vi "Start Discovery Service.vi"(8 "error in":errorcluster, 11 "key file path":path) -> (0 "error out":errorcluster)   [LabVIEW 2020, in "MeasurementLink Discovery.lvlib"]
doc: "This VI starts the MeasurementLink.DiscoveryService.exe."
uses:
  <vilib>/Utility/sysdir.llb/System Directory Type.ctl
  MeasurementLink Measurement Server/Helpers/Error Strings Global Internal.vi
  <vilib>/ErrorRing/Error Ring.xnode
  MeasurementLink Discovery.lvlib
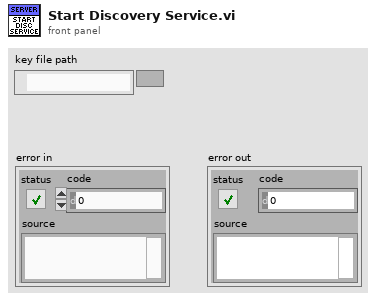
[diagram p1: front panel]
types:
  T1 = enum16{"open", "replace", "create", "open or create", "replace or create", "replace or create with confirmation"}
  T2 = typedef "System Directory Type.ctl" = i32
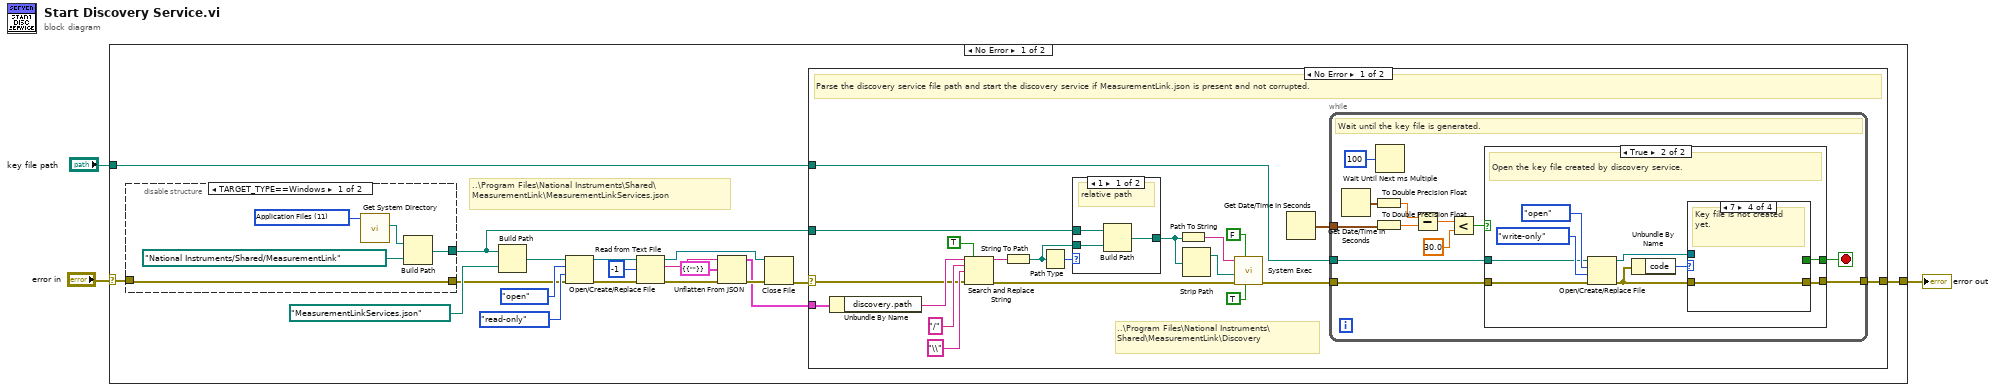
[diagram p0: block diagram]
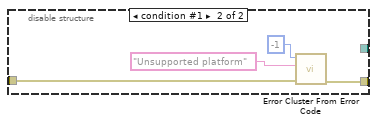
[diagram p2: hidden frame]
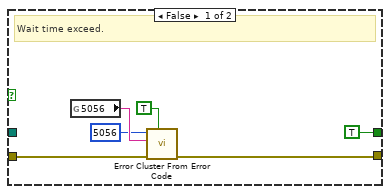
[diagram p4: hidden frame]
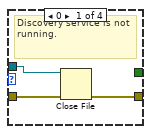
[diagram p5: hidden frame]
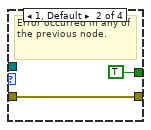
[diagram p6: hidden frame]
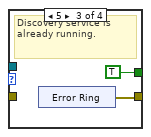
[diagram p7: hidden frame]
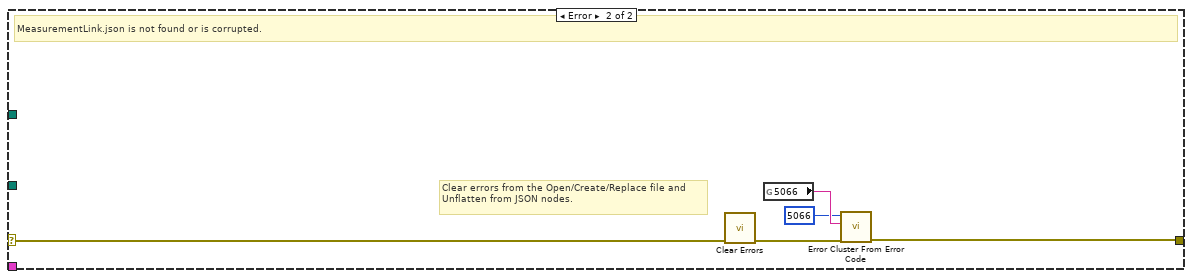
[diagram p8: hidden frame]
diagram:
  n1 = case shown="No Error" "error in" {
    selector: "error in" -> [w17 w97]
    tunnel: [w16 w97] -> w2
    tunnel: "key file path" -> [w15 _]
    frame No Error {
      # "..\\Program Files\\National Instruments\\Shared\\MeasurementLink\\MeasurementLinkServices.json"
      n2 = disable-structure shown="TARGET_TYPE==Windows" {
        disable-tunnel: [w24 _] -> w14
        disable-tunnel: w17 -> [w23 w29]
        disable-tunnel: [w23 w28] -> w18
        frame condition #0 (active) {
          w27 = T2 11 items=["User Home"=0, "User Desktop"=1, "User Documents"=2, "User Application Data"=3, "User Preferences"=4, "User Temporary"=5, "Public Documents"=6, "Public Application Data"=7, "Public Preferences"=8, "Public Cache"=13, "System Core Libraries"=9, "System Installed Libraries"=10, "Application Files"=11, "Boot Volume Root"=12] ("system directory type")
          n3 = call <vilib>:"Get System Directory.vi"("system directory type"=w27) -> ("system directory"=w26:path)  [unwired: 10 in]
          n4 = Build Path(base path=w26, name or relative path=path "National Instruments/Shared/MeasurementLink") -> (appended path=w24:path)
        }
        frame condition #1 {
          n5 = call <vilib>:"Error Cluster From Error Code.vi"("error in (no error)"=w29, "error message (\"\")"="Unsupported platform" ("error message (\"\")"), "error code (0)"=-1) -> ("error out"=w28:errorcluster)  [unwired: 6 in]
        }
      }
      n6 = Build Path(base path=w14, name or relative path=path "MeasurementLinkServices.json") -> (appended path=w21:path)
      n7 = Open/Create/Replace File(file path (use dialog)=w21, error in=w18, operation (0:open)=T1."open", access (0:read/write)=enum16{"read/write", "read-only", "write-only"}."read-only") -> (refnum out=w6:refnum<file>, error out=w9:errorcluster)  [unwired: 2 in, 1 out]
      n8 = Read from Text File(file (use dialog)=w6, count=-1, error in=w9) -> (refnum out=w7:refnum<file>, text=w11:string, error out=w13:errorcluster)  [unwired: 1 in, 1 out]
      n9 = Unflatten From JSON(JSON string=w11, type and defaults=cluster{"discovery":cluster{"path":string}} {"discovery"={"path"=""}}, error in (no error)=w13) -> (value=w4:cluster{"discovery":cluster{"path":string}}, error out=w8:errorcluster)  [unwired: 4 in]
      n10 = Close File(refnum=w7, error in=w8) -> (error out=w5:errorcluster)  [unwired: 1 out]
      n11 = case shown="No Error" w5 {
        selector: w5 -> [w33 w96]
        tunnel: [w41 w94] -> w16
        tunnel: w15 -> [w40 _]
        tunnel: w14 -> [w36 _]
        tunnel: w4 -> [w32 _]
        frame No Error {
          # "..\\Program Files\\National Instruments\\Shared\\MeasurementLink\\Discovery"
          # "Parse the discovery service file path and start the discovery service if MeasurementLink.json is present and not corrupted."
          n12 = Unbundle By Name(w32) -> ("discovery.path"=w34:string)
          n13 = Search and Replace String(replace all?=TRUE ("replace all? (F)"), input string=w34, search string="/", replace string="\\" ("replace string (\"\")"), error in=w33) -> (result string=w37:string, error out=w47:errorcluster)  [unwired: 3 in, 2 out]
          n14 = String To Path(string=w37) -> (path=w38:path)
          n15 = Path Type(1:w38) -> (0:w39:i16)
          n16 = case shown="1" w39 {
            tunnel: [w54 w55] -> w35
            tunnel: w36 -> [w53 _]
            tunnel: w38 -> [w52 w55]
            frame 1 {
              # "relative path"
              n17 = Build Path(base path=w53, name or relative path=w52) -> (appended path=w54:path)
            }
            frame Default {
              # "absolute path"
            }
          }
          n18 = Path To String(path=w35) -> (string=w48:string)
          n19 = Strip Path(path=w35) -> (stripped path=w49:path)  [unwired: 1 out]
          n20 = call <vilib>:"System Exec.vi"("run minimized? (F)"=TRUE, "wait until completion? (T)"=FALSE, "error in (no error)"=w47, "working directory"=w49, "command line"=w48) -> ("error out"=w43:errorcluster)  [unwired: 3 in, 3 out]
          n21 = Get Date/Time In Seconds() -> (seconds since 1Jan1904=w44:timestamp)
          n22 = while {
            tunnel: w43 -> [w64]
            tunnel: w40 -> [w65]
            tunnel: [w62] -> w41
            tunnel: w44 -> [w57]
            stop <- w63 stop-if-true
            # "Wait until the key file is generated."
            n23 = Get Date/Time In Seconds() -> (seconds since 1Jan1904=w58:timestamp)
            n24 = To Double Precision Float(number=w58) -> (double precision float=w59:dbl)
            n25 = To Double Precision Float(number=w57) -> (double precision float=w56:dbl)
            n26 = Wait Until Next ms Multiple(millisecond multiple=u32 100) -> ()  [unwired: 1 out]
            n27 = Subtract(x=w59, y=w56) -> (x-y=w60:dbl)
            n28 = Less?(x=w60, y=30.0) -> (x < y?=w67:bool)
            n29 = case shown="True" w67 {
              tunnel: w65 -> [_ w79]
              tunnel: w64 -> [w69 w80]
              tunnel: [TRUE w75] -> w63
              tunnel: [w68 w76] -> w62
              frame False {
                # "Wait time exceed."
                n30 = global read "Error Strings Global Internal.vi" "5056"() -> (w72:string)
                n31 = call <vilib>:"Error Cluster From Error Code.vi"("show call chain? (False)"=TRUE, "error in (no error)"=w69, "error message (\"\")"=w72, "error code (0)"=5056) -> ("error out"=w68:errorcluster)  [unwired: 5 in]
              }
              frame True {
                # "Open the key file created by discovery service."
                n32 = Open/Create/Replace File(file path (use dialog)=w79, error in=w80, operation (0:open)=T1."open", access (0:read/write)=enum16{"read/write", "read-only", "write-only"}."write-only") -> (refnum out=w74:refnum<file>, error out=w77:errorcluster)  [unwired: 2 in, 1 out]
                n33 = Unbundle By Name(w77) -> ("code"=w78:i32)
                n34 = case shown="7" w78 {
                  tunnel: [w84 w87 w89 w91] -> w76
                  tunnel: w77 -> [w85 w87 _ w91]
                  tunnel: [_ TRUE TRUE _] -> w75
                  tunnel: w74 -> [w83 _ _ _]
                  frame 0 {
                    # "Discovery service is not running."
                    n35 = Close File(refnum=w83, error in=w85) -> (error out=w84:errorcluster)  [unwired: 1 out]
                  }
                  frame 1, Default {
                    # "Error occurred in any of the previous node."
                  }
                  frame 5 {
                    # "Discovery service is already running."
                    n36 = xnode "Error Ring"() -> ("error out"=w89:errorcluster)
                  }
                  frame 7 {
                    # "Key file is not created yet."
                  }
                }
              }
            }
          }
        }
        frame Error {
          # "Clear errors from the Open/Create/Replace file and Unflatten from JSON nodes."
          # "MeasurementLink.json is not found or is corrupted."
          n37 = call <vilib>:"Clear Errors.vi"("error in (no error)"=w96) -> ("error out"=w95:errorcluster)  [unwired: 5 in, 1 out]
          n38 = global read "Error Strings Global Internal.vi" "5066"() -> (w93:string)
          n39 = call <vilib>:"Error Cluster From Error Code.vi"("error in (no error)"=w95, "error message (\"\")"=w93, "error code (0)"=5066) -> ("error out"=w94:errorcluster)  [unwired: 6 in]
        }
      }
    }
    frame Error {
    }
  }
  "error out" <- w2
